vi "Reset Table.vi"(8 "error in (no error)":errorcluster, 11 "Result Table.lvclass":refnum<class "Result Table V2.lvclass">) -> (0 "error out":errorcluster, 3 "Result Table":refnum<class "Result Table V2.lvclass">)   [LabVIEW 2020, in "Result Table V2.lvclass"]
uses:
  Result Table V2.lvclass
  Result Table V2.lvclass/Result Table V2.ctl
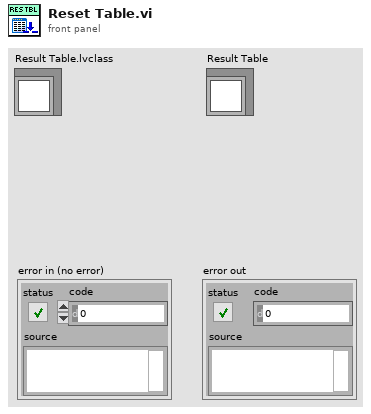
[diagram p1: front panel]
types:
  T1 = typedef "Result Table V2.lvclass/Results.ctl" = cluster{"Method Count":u32, "Executed Methods":u32, "Passed Methods":u32, "Failed Methods":u32, "Method Errors":u32, "Skipped Method":u32}
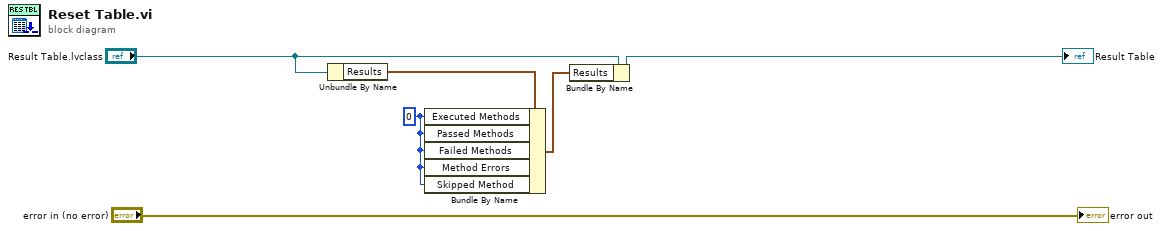
[diagram p0: block diagram]
diagram:
  w2 = u32 0 ("Executed Methods")
  n1 = Unbundle By Name("Result Table.lvclass") -> ("Results"=w3:T1)
  n2 = Bundle By Name(cluster=w3, "Executed Methods"=w2, "Passed Methods"=w2, "Failed Methods"=w2, "Method Errors"=w2, "Skipped Method"=w2) -> (w1:T1)
  n3 = Bundle By Name(cluster="Result Table.lvclass", "Results"=w1) -> (→"Result Table":refnum<class "Result Table V2.lvclass">)
  "error out" <- "error in (no error)"
